vi "FT10_M4X Find Vertical Range.vi"(11 "Sample":sgl[](array[numeric])) -> (3 "Range":T1(ring))   [LabVIEW 2024]
doc: "Copy of \"Find Vertical Range.vi\" from HWT_Lillis_7854.lvproj"
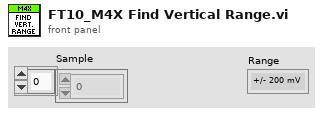
[diagram p1: front panel]
types:
  T1 = enum16{"+/- 200 mV", "+/- 500 mV", "+/- 1 V", "+/- 2 V", "+/- 5 V", "+/- 10 V"}
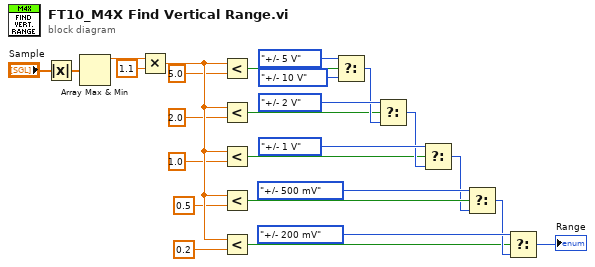
[diagram p0: block diagram]
diagram:
  n1 = Absolute Value(x="Sample") -> (abs(x)=w25:sgl[])
  n2 = Array Max & Min(array=w25) -> (max value=w26:sgl)  [unwired: 3 out]
  n3 = Multiply(x=w26, y=1.1) -> (x*y=w14:dbl)
  n4 = Less?(x=w14, y=5.0) -> (x < y?=w3:bool)
  n5 = Less?(x=w14, y=2.0) -> (x < y?=w5:bool)
  n6 = Less?(x=w14, y=1.0) -> (x < y?=w8:bool)
  n7 = Less?(x=w14, y=0.5) -> (x < y?=w12:bool)
  n8 = Less?(x=w14, y=0.2) -> (x < y?=w15:bool)
  n9 = Select(t=T1."+/- 5 V" ("Range"), s=w3, f=T1."+/- 10 V" ("Range")) -> (s? t:f=w6:T1)
  n10 = Select(t=T1."+/- 2 V" ("Range"), s=w5, f=w6) -> (s? t:f=w9:T1)
  n11 = Select(t=T1."+/- 1 V" ("Range"), s=w8, f=w9) -> (s? t:f=w10:T1)
  n12 = Select(t=T1."+/- 500 mV" ("Range"), s=w12, f=w10) -> (s? t:f=w16:T1)
  n13 = Select(t=T1."+/- 200 mV" ("Range"), s=w15, f=w16) -> (s? t:f=→"Range":T1)
